vi "JSON Array To String.vi"(7 "enable LabVIEW extensions? (T)":bool=TRUE, 8 "error in (no error)":errorcluster, 11 "JSON Array in":refnum<class "JSON Helper.lvclass">) -> (0 "error out":errorcluster, 3 "String":string)   [LabVIEW 2016, in "JSON Helper.lvclass"]
doc: "Flattens the given JSON data to a string."
uses:
  JSON Helper/JSON Helper.lvclass
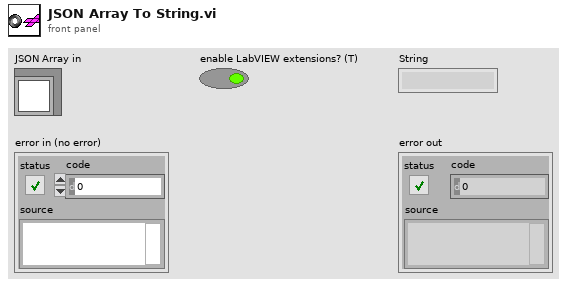
[diagram p1: front panel]
types:
  T1 = typedef "JSON Helper.lvclass/JSON Types.ctl" = enum16{"String", "Numeric", "Boolean", "NULL", "Object", "Array"}
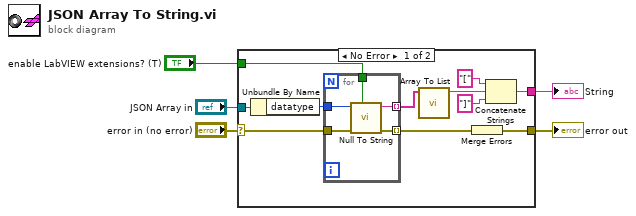
[diagram p0: block diagram]
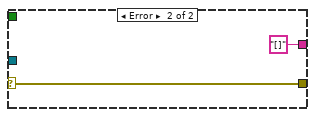
[diagram p2: hidden frame]
diagram:
  n1 = case shown="No Error" "error in (no error)" {
    selector: "error in (no error)" -> [w14 w23]
    tunnel: "JSON Array in" -> [w16 _]
    tunnel: [w12 w23] -> w3
    tunnel: [w11 "[]"] -> w2
    tunnel: "enable LabVIEW extensions? (T)" -> [w6 _]
    frame No Error {
      n2 = Unbundle By Name(w16) -> ("datatype"=w7:T1)
      n3 = for {
        tunnel: [w21] -> w15 mode=indexing
        tunnel: w14 -> [w20]
        tunnel: [w19] -> w13 mode=indexing
        tunnel: w7 -> [w18]
        tunnel: w6 -> [w17]
        n4 = call "Null To String.vi"("enable LabVIEW extensions? (T)"=w17, "error in (no error)"=w20, "JSON Datatype in"=w18) -> ("error out"=w19:errorcluster, "String"=w21:string)  [unwired: 7 in]
      }
      n5 = call "Array To List.vi"("Array"=w15) -> ("String"=w10:string)  [unwired: 10 in]
      n6 = Merge Errors(w13) -> (w12:errorcluster)
      n7 = Concatenate Strings("[" ("string"), w10, "]" ("string")) -> (w11:string)
    }
    frame Error {
    }
  }
  "String" <- w2
  "error out" <- w3
